vi "Multi-socket Data Generation.vi"() -> ()   [LabVIEW 2009]
panel:
  out "subarray 2":string[](array[string])
  out "subarray":string[](array[string])
  out "Multi Socket Data Out":string[][](array[string])
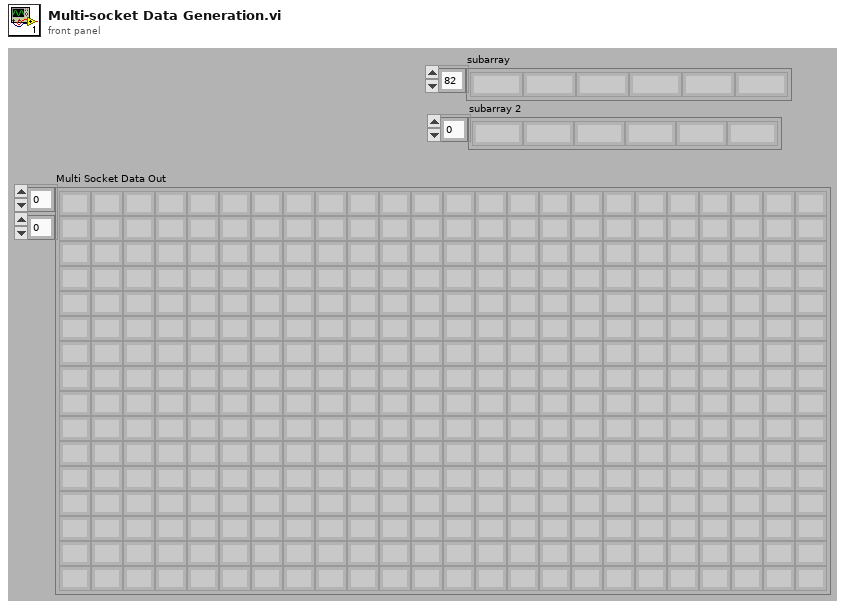
[diagram p1: front panel]
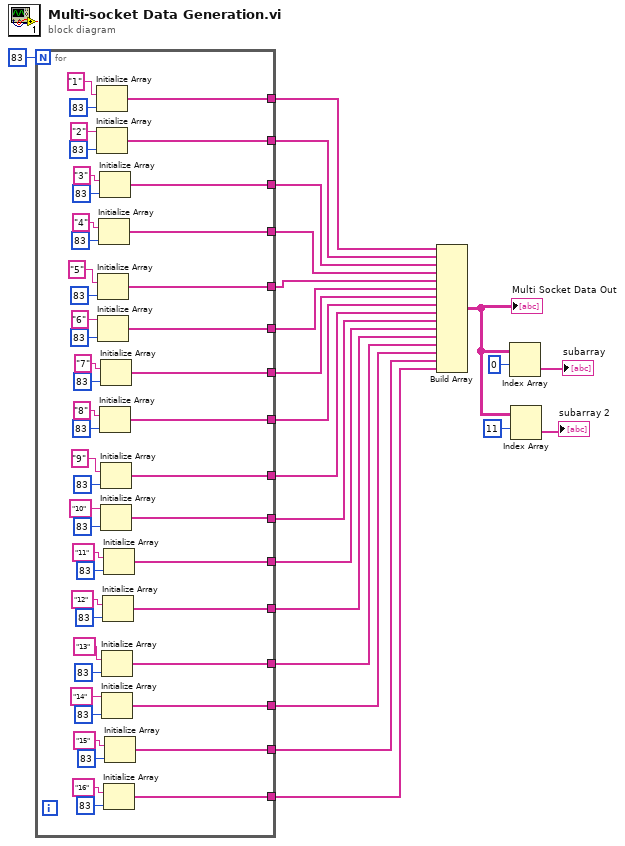
[diagram p0: block diagram]
diagram:
  n1 = for {
    N: 83 -> [_]
    tunnel: [w60] -> w21
    tunnel: [w67] -> w20
    tunnel: [w62] -> w19
    tunnel: [w61] -> w18
    tunnel: [w42] -> w17
    tunnel: [w41] -> w16
    tunnel: [w40] -> w15
    tunnel: [w39] -> w14
    tunnel: [w38] -> w13
    tunnel: [w37] -> w12
    tunnel: [w36] -> w11
    tunnel: [w35] -> w10
    tunnel: [w26] -> w4
    tunnel: [w25] -> w3
    tunnel: [w24] -> w2
    tunnel: [w23] -> w1
    n2 = Initialize Array("1", 83 ("dimension size")) -> (w60:string[])
    n3 = Initialize Array("2" ("element"), 83 ("dimension size")) -> (w67:string[])
    n4 = Initialize Array("5", 83 ("dimension size")) -> (w42:string[])
    n5 = Initialize Array("6" ("element"), 83 ("dimension size")) -> (w41:string[])
    n6 = Initialize Array("4" ("element"), 83 ("dimension size")) -> (w61:string[])
    n7 = Initialize Array("3" ("element"), 83 ("dimension size")) -> (w62:string[])
    n8 = Initialize Array("8" ("element"), 83 ("dimension size")) -> (w39:string[])
    n9 = Initialize Array("7" ("element"), 83 ("dimension size")) -> (w40:string[])
    n10 = Initialize Array("9", 83 ("dimension size")) -> (w38:string[])
    n11 = Initialize Array("10" ("element"), 83 ("dimension size")) -> (w37:string[])
    n12 = Initialize Array("13", 83 ("dimension size")) -> (w26:string[])
    n13 = Initialize Array("14" ("element"), 83 ("dimension size")) -> (w25:string[])
    n14 = Initialize Array("12" ("element"), 83 ("dimension size")) -> (w35:string[])
    n15 = Initialize Array("11" ("element"), 83 ("dimension size")) -> (w36:string[])
    n16 = Initialize Array("16" ("element"), 83 ("dimension size")) -> (w23:string[])
    n17 = Initialize Array("15" ("element"), 83 ("dimension size")) -> (w24:string[])
  }
  n18 = Build Array(w21, w20, w19, w18, w17, w16, w15, w14, w13, w12, w11, w10, w4, w3, w2, w1) -> (w7:string[][])
  "Multi Socket Data Out" <- w7
  n19 = Index Array(array=w7, index (row)=0) -> (element=→"subarray":string[])  [unwired: 1 in]
  n20 = Index Array(array=w7, index (row)=11) -> (element=→"subarray 2":string[])  [unwired: 1 in]
